vi "Label Connected Components 2D.vi"(0 "Array":bool[][](array[boolean]), 1 "Connectivity (8)":enum16{"4", "8"}(ring)=enum."8") -> (2 "Intensity Graph":i32[][](graph), 3 "N Labels":i32)   [LabVIEW 2020, in "VIM Tools.lvlib"]
uses:
  VIM Tools.lvlib
  a131e0ae-e03b-4dbc-9548-a14009ba621e.vi
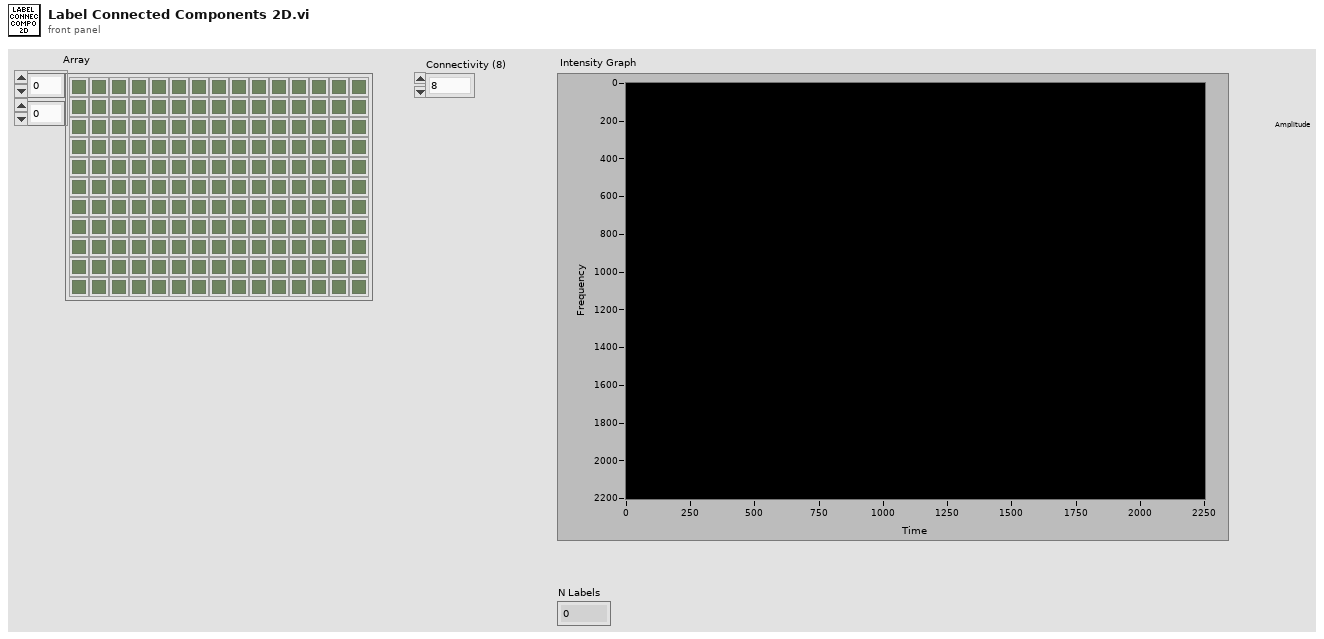
[diagram p1: front panel]
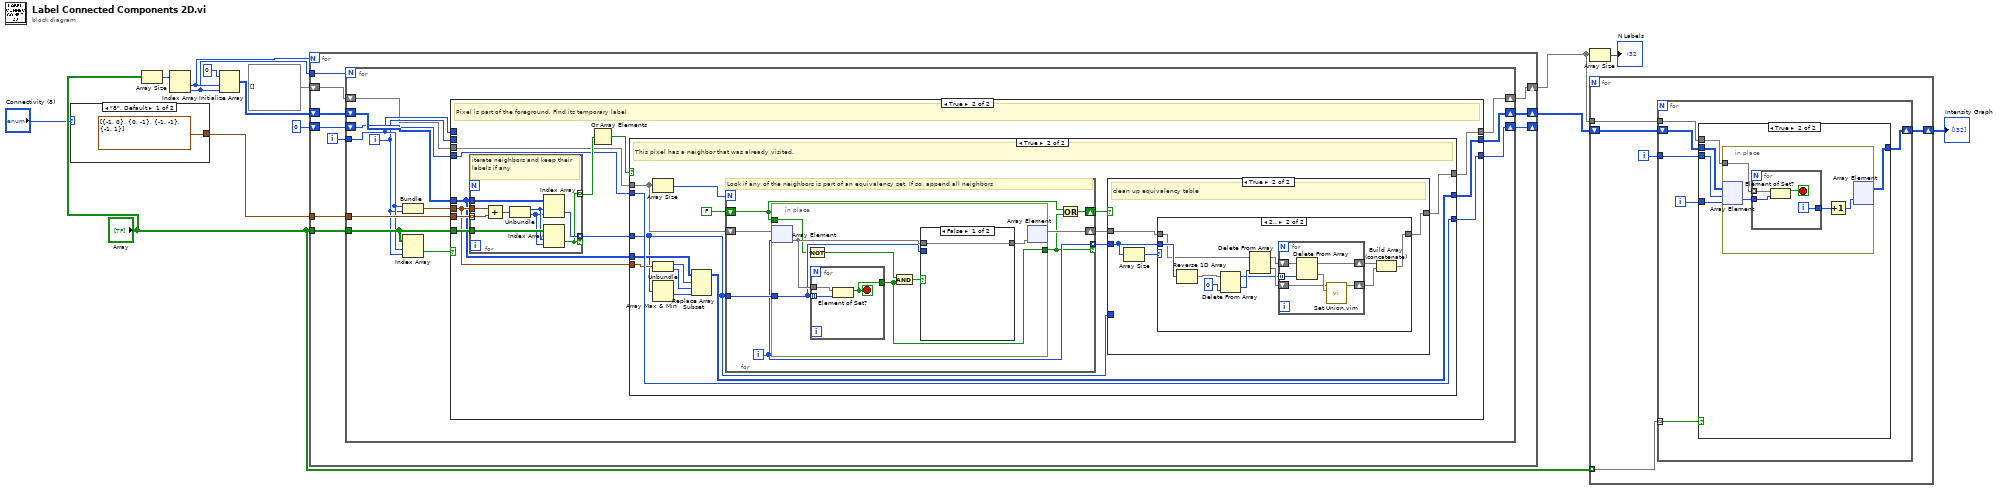
[diagram p0: block diagram]
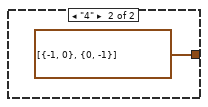
[diagram p2: hidden frame]
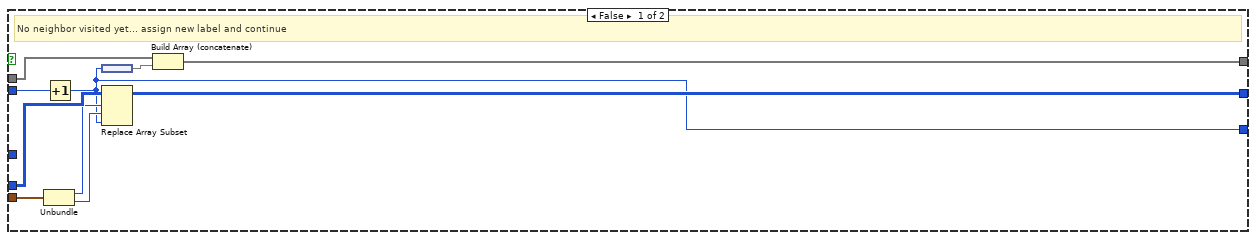
[diagram p5: hidden frame]
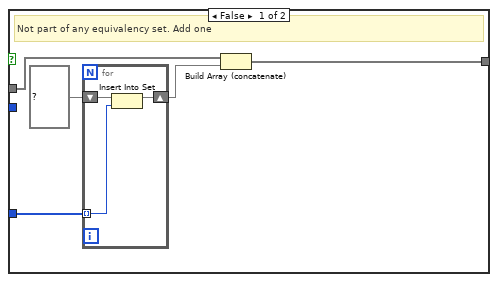
[diagram p6: hidden frame]
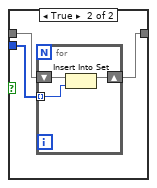
[diagram p8: hidden frame]
diagram:
  n1 = case shown="\"8\", Default" "Connectivity (8)" {
    tunnel: [cluster{i32, i32}[] [{-1, 0}, {0, -1}, {-1, -1}, {-1, 1}] cluster{i32, i32}[] [{-1, 0}, {0, -1}]] -> w11
    frame "8", Default {
    }
    frame "4" {
    }
  }
  n2 = Array Size(array="Array") -> (size(s)=w14:i32[])
  n3 = Index Array(array=w14) -> (element #1=w9:i32, element #2=w8:i32)  [unwired: 2 in]
  n4 = Initialize Array(0, w9, w8) -> (w12:i32[][])
  n5 = for {
    N: w9 -> [_]
    tunnel: "Array" -> [w26]
    shift-right: [w24] -> w6
    shift-left: w12 -> [w25]
    tunnel: w11 -> [w23]
    shift-right: [w20] -> _
    shift-left: 0 -> [w21]
    tunnel: w8 -> [w19]
    shift-right: [w17] -> w2
    shift-left: set{i32}[] [] ("Array") -> [w18]
    i -> [w22]
    n6 = for {
      N: w19 -> [_]
      tunnel: w26 -> [w36]
      shift-right: [w33] -> w24
      shift-left: w25 -> [w35]
      tunnel: w23 -> [w37]
      tunnel: w22 -> [w31]
      shift-right: [w32] -> w20
      shift-left: w21 -> [w34]
      shift-right: [w28] -> w17
      shift-left: w18 -> [w27]
      i -> [w30]
      n7 = Bundle(w31, w30) -> (w29:cluster{i32, i32})  [unwired: 1 in]
      n8 = Index Array(array=w36, index (row)=w31, index (col)=w30) -> (element=w38:bool)
      n9 = case shown="True" w38 {
        tunnel: w37 -> [_ w47]
        tunnel: w36 -> [_ w53]
        tunnel: w35 -> [w41 w45]
        tunnel: w34 -> [w40 w50]
        tunnel: [w41 w49] -> w33
        tunnel: w31 -> [_ _]
        tunnel: w30 -> [_ _]
        tunnel: [w40 w48] -> w32
        tunnel: w29 -> [_ w46]
        tunnel: [w39 w42] -> w28
        tunnel: w27 -> [w39 w43]
        frame False {
        }
        frame True {
          # "Pixel is part of the foreground. Find its temporary label"
          n10 = for {
            tunnel: w53 -> [w141]
            tunnel: w47 -> [w140] mode=indexing
            tunnel: [w133] -> w52 mode=indexing
            tunnel: w46 -> [w138]
            tunnel: w45 -> [w135]
            tunnel: [w134] -> w44 mode=indexing if=w133
            # "iterate neighbors and keep their labels if any"
            n11 = Add(x=w138, y=w140) -> (x+y=w139:cluster{i32, i32})
            n12 = Unbundle(w139) -> (w137:i32, w136:i32)
            n13 = Index Array(array=w135, index (row)=w137, index (col)=w136) -> (element=w134:i32)
            n14 = Index Array(array=w141, index (row)=w137, index (col)=w136) -> (element=w133:bool)
          }
          n15 = Or Array Elements(Boolean array=w52) -> (logical OR=w51:bool)
          n16 = case shown="True" w51 {
            tunnel: w50 -> [w61 w77]
            tunnel: w45 -> [w63 w75]
            tunnel: [w62 w78] -> w49
            tunnel: [w56 w77] -> w48
            tunnel: w46 -> [w60 w76]
            tunnel: w44 -> [_ w67]
            tunnel: [w55 w68] -> w42
            tunnel: w43 -> [w57 w70]
            frame False {
              # "No neighbor visited yet... assign new label and continue"
              n17 = Unbundle(w60) -> (w59:i32, w58:i32)
              n18 = Increment(x=w61) -> (x+1=w56:i32)
              n19 = node(w56) -> (w54:set{i32})
              n20 = Replace Array Subset(array=w63, new element=w56, index (row)=w59, index (col)=w58) -> (w62:i32[][])
              n21 = Build Array (concatenate)(w57, w54) -> (w55:set{i32}[])
            }
            frame True {
              # "This pixel has a neighbor that was already visited."
              n22 = Array Size(array=w70) -> (size(s)=w71:i32)
              n23 = Unbundle(w76) -> (w74:i32, w73:i32)
              n24 = Array Max & Min(array=w67) -> (min value=w72:i32)  [unwired: 3 out]
              n25 = Replace Array Subset(array=w75, new element=w72, index (row)=w74, index (col)=w73) -> (w78:i32[][])
              n26 = for {
                N: w71 -> [_]
                shift-right: [w114] -> w69
                shift-left: w70 -> [w115]
                tunnel: w67 -> [w113]
                tunnel: [w112] -> w65 mode=indexing if=w110
                shift-right: [w111] -> w64
                shift-left: FALSE -> [w109]
                i -> [w112]
                # "Look if any of the neighbors is part of an equivalency set. If so, append all neighbors"
                n27 = in-place {
                  in-place-border: w113 -> [w119]
                  in-place-border: [w121] -> w110
                  in-place-border: w109 -> [w117]
                  n28 = in-place-array #1(w115, w112) -> (w120:set{i32})
                  n29 = Not(x=w117) -> (.not. x?=w116:bool)
                  n30 = for {
                    tunnel: w119 -> [w132] mode=indexing
                    tunnel: w120 -> [w131]
                    tunnel: [w130] -> w121
                    stop <- w130 stop-if-true
                    n31 = Element of Set?(10:w132, 11:w131) -> (3:w130:bool)
                  }
                  n32 = And(x=w116, y=w121) -> (x .and. y?=w118:bool)
                  n33 = case shown="False" w118 {
                    tunnel: [w123 w126] -> w122
                    tunnel: w120 -> [w123 w125]
                    tunnel: w119 -> [_ w124]
                    frame False {
                    }
                    frame True {
                      n34 = for {
                        shift-right: [w128] -> w126
                        shift-left: w125 -> [w129]
                        tunnel: w124 -> [w127] mode=indexing
                        n35 = Insert Into Set(10:w127, 11:w129) -> (3:w128:set{i32})  [unwired: 1 out]
                      }
                    }
                  }
                  n36 = in-place-array #1(w122) -> (w114:set{i32}[])  [unwired: 1 out]
                }
                n37 = Or(x=w109, y=w110) -> (x .or. y?=w111:bool)
              }
              n38 = case shown="True" w64 {
                tunnel: [w81 w89] -> w68
                tunnel: w69 -> [w83 w88]
                tunnel: w67 -> [w79 _]
                tunnel: w65 -> [_ w87]
                frame False {
                  # "Not part of any equivalency set. Add one"
                  n39 = for {
                    shift-right: [w85] -> w80
                    shift-left: set{i32} {} ("element") -> [w86]
                    tunnel: w79 -> [w84] mode=indexing
                    n40 = Insert Into Set(10:w84, 11:w86) -> (3:w85:set{i32})  [unwired: 1 out]
                  }
                  n41 = Build Array (concatenate)(w83, w80) -> (w81:set{i32}[])
                }
                frame True {
                  # "clean up equivalency table"
                  n42 = Array Size(array=w87) -> (size(s)=w90:i32)
                  n43 = case shown="2.." w90 {
                    tunnel: [w91 w93] -> w89
                    tunnel: w88 -> [w91 w100]
                    tunnel: w87 -> [_ w101]
                    frame 0, Default {
                    }
                    frame 2.. {
                      n44 = Reverse 1D Array(array=w101) -> (reversed array=w102:i32[])
                      n45 = Delete From Array(array=w102, index=0) -> (deleted portion=w99:i32, array with subset deleted=w96:i32[])  [unwired: 1 in]
                      n46 = Delete From Array(array=w100, index=w99) -> (deleted portion=w98:set{i32}, array with subset deleted=w97:set{i32}[])  [unwired: 1 in]
                      n47 = for {
                        shift-right: [w107] -> w94
                        shift-left: w97 -> [w108]
                        shift-right: [w104] -> w95
                        shift-left: w98 -> [w105]
                        tunnel: w96 -> [w103] mode=indexing
                        n48 = Delete From Array(array=w108, index=w103) -> (deleted portion=w106:set{i32}, array with subset deleted=w107:set{i32}[])  [unwired: 1 in]
                        n49 = call "Set Union.vim"("set 2"=w106, "set 1"=w105) -> ("union"=w104:set{i32})  [unwired: 9 in]
                      }
                      n50 = Build Array (concatenate)(w94, w95) -> (w93:set{i32}[])
                    }
                  }
                }
              }
            }
          }
        }
      }
    }
  }
  n51 = Array Size(array=w2) -> (size(s)=→"N Labels":i32)
  n52 = for {
    shift-right: [w145] -> w4
    shift-left: w6 -> [w146]
    tunnel: w2 -> [w144]
    tunnel: "Array" -> [w142] mode=indexing
    i -> [w143]
    n53 = for {
      shift-right: [w147] -> w145
      shift-left: w146 -> [w152]
      tunnel: w144 -> [w148]
      tunnel: w143 -> [w151]
      tunnel: w142 -> [w149] mode=indexing
      i -> [w150]
      n54 = case shown="True" w149 {
        tunnel: w152 -> [w153 w158]
        tunnel: w151 -> [_ w155]
        tunnel: w150 -> [_ w154]
        tunnel: w148 -> [_ w156]
        tunnel: [w153 w157] -> w147
        frame False {
        }
        frame True {
          n55 = in-place {
            in-place-border: w156 -> [w162]
            n56 = in-place-array #2(w158, w155, w154) -> (w161:i32)
            n57 = for {
              tunnel: w162 -> [w166] mode=indexing
              tunnel: w161 -> [w165]
              tunnel: [w163] -> w160
              i -> [w163]
              stop <- w164 stop-if-true
              n58 = Element of Set?(10:w165, 11:w166) -> (3:w164:bool)
            }
            n59 = Increment(x=w160) -> (x+1=w159:i32)
            n60 = in-place-array #2(w159) -> (w157:i32[][])  [unwired: 2 out]
          }
        }
      }
    }
  }
  "Intensity Graph" <- w4
